vi "Get Configuration.vi"(8 "error in (no error)":errorcluster, 11 "UDP Transfer Rx Configuration in":refnum<class "UDP Transfer Rx Configuration.lvclass">) -> (0 "error out":errorcluster, 2 "transfer settings":T1, 3 "UDP Transfer Rx Configuration out":refnum<class "UDP Transfer Rx Configuration.lvclass">)   [LabVIEW 2017, in "DSF Core.lvlib" / "UDP Transfer Rx Configuration.lvclass"]
uses:
  UDP Transfer Rx Configuration.lvclass
  Rx Transfer Settings.ctl
  UDP Transfer Rx Configuration.lvclass/UDP Transfer Rx Configuration.ctl
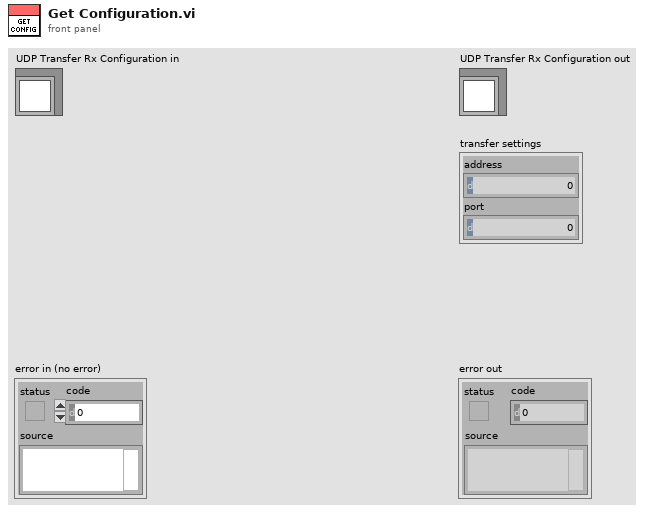
[diagram p1: front panel]
types:
  T1 = typedef "DSF Core.lvlib/UDP Transfer Rx Configuration.lvclass/Rx Transfer Settings.ctl" = cluster{"address":u32, "port":u16}
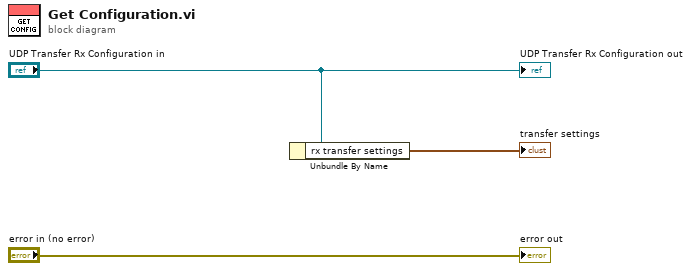
[diagram p0: block diagram]
diagram:
  n1 = Unbundle By Name("UDP Transfer Rx Configuration in") -> ("rx transfer settings"=→"transfer settings":T1)
  "error out" <- "error in (no error)"
  "UDP Transfer Rx Configuration out" <- "UDP Transfer Rx Configuration in"
